vi "Plot Multi-XY_modded.vi"(0 "picture":picture, 1 "desired font(Application)":T6(ring)=enum."Application Font", 3 "[user-specified font]":T7, 5 "data":cluster{"data":cluster{"x":dbl, "y":dbl}[]}[](array[cluster]) {"data"."y" format="%0.2f"; "data"."x" format="%0.2f"}, 7 "dimensions (w,h)":cluster{"width":i16, "height":i16}, 9 "line style":T1={"Width"=1, "Style"=enum."Solid"}, 11 "top left point(0, 0)":cluster{"x":i16, "y":i16}, 12 "cartesian axis attributes":T8={"x minimum"=0.0, "x maximum"=0.0, "x log?"=FALSE, "x precision"=1, "x format"=enum."Decimal", "y minimum"=0.0, "y maximum"=0.0, "y log?"=FALSE, "y precision"=1, "y format"=enum."Decimal"} {"x minimum" format="%0.2f"; "x maximum" format="%0.2f"; "y minimum" format="%0.2f"; "y maximum" format="%0.2f"}, 13 "cartesian grid cosmetics":T3={"line color"=39168, "text color"=65280, "tick length(3)"=3, "crossing axes"=FALSE, "visible grid?"=TRUE}, 14 "XY plot cosmetics":T5(array[cluster])=[{"plot color"=16776960, "XY plot type"=enum."sized scatter plot", "baseline"=0.0}, {"plot color"=65280, "XY plot type"=enum."connected points", "baseline"=0.0}, {"plot color"=65535, "XY plot type"=enum."connected points", "baseline"=0.0}] {"baseline" format="%0.2f"}, 15 "[sized scatter plot cosmetics]":T2(array[cluster])=[{"min size"=1, "max size"=5, "maps to max size"=5, "color array"=[16776960, 65280, 16711680, 255]}]) -> (4 "new picture":picture)   [LabVIEW 2018]
doc: "Takes a picture and an array of plots and appends a picture of an XY graph of the data with the plots overlaid on the same graph."
uses:
  <vilib>/picture/cartesn2.llb/XY Plot Type.ctl
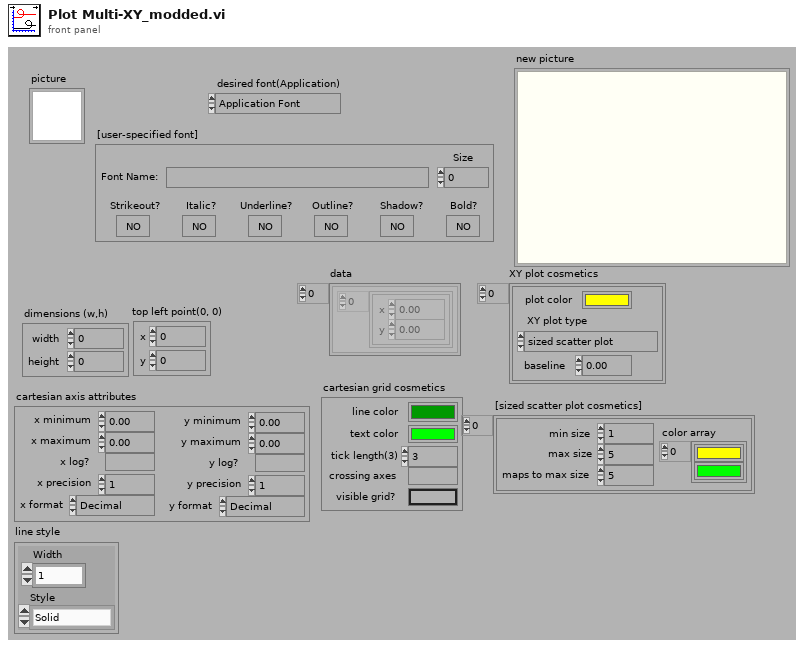
[diagram p1: front panel]
types:
  T1 = cluster{"Width":u16, "Style":enum32{"Solid", "Dash", "Dot", "DashDot", "DashDotDot"}}
  T2 = cluster{"min size":i16, "max size":i16, "maps to max size":i16, "color array":u32[]}[]
  T3 = cluster{"line color":u32, "text color":u32, "tick length(3)":i16, "crossing axes":bool, "visible grid?":bool}
  T4 = typedef "XY Plot Type.ctl" = enum16{"points", "squares", "circles", "connected points", "connected squares", "connected circles", "comb plot", "sized scatter plot", "sized-colored scatter plot", "min-max lines"}
  T5 = cluster{"plot color":u32, "XY plot type":T4, "baseline":dbl}[]
  T6 = enum16{"User-specified Font", "Application Font", "System Font", "Dialog Font"}
  T7 = cluster{"Font Name:":string, "Size":i16, "Strikeout?":bool, "Italic?":bool, "Underline?":bool, "Outline?":bool, "Shadow?":bool, "Bold?":bool}
  T8 = cluster{"x minimum":dbl, "x maximum":dbl, "x log?":bool, "x precision":u8, "x format":enum8{"Decimal", "Scientific", "Engineering", "Binary", "Octal", "Hex", "Timestamp"}, "y minimum":dbl, "y maximum":dbl, "y log?":bool, "y precision":u8, "y format":enum8{"Decimal", "Scientific", "Engineering", "Binary", "Octal", "Hex", "Timestamp"}}
  T9 = cluster{"left":i16, "top":i16, "right":i16, "bottom":i16}
  T10 = cluster{"plot color":u32, "XY plot type":T4, "baseline":dbl}
  T11 = cluster{"min size":i16, "max size":i16, "maps to max size":i16, "color array":u32[]}
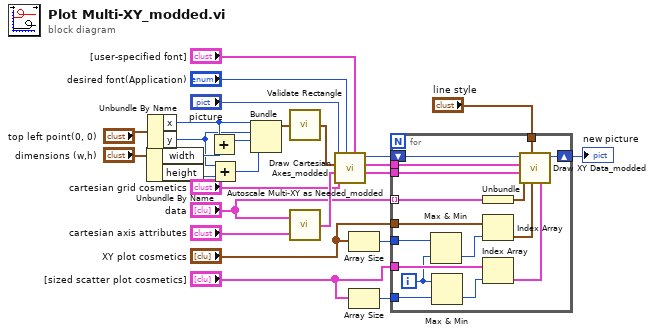
[diagram p0: block diagram]
diagram:
  n1 = Unbundle By Name("dimensions (w,h)") -> ("width"=w10:i16, "height"=w9:i16)
  n2 = Unbundle By Name("top left point(0, 0)") -> ("x"=w8:i16, "y"=w7:i16)
  n3 = Add(x=w8, y=w10) -> (x+y=w6:i16)
  n4 = Add(x=w7, y=w9) -> (x+y=w5:i16)
  n5 = Bundle("x"=w8, "y"=w7, w6, w5) -> (w2:cluster{"x":i16, "y":i16, i16, i16})  [unwired: 1 in]
  n6 = call <vilib>:"Validate Rectangle.vi"("rect"=w2) -> ("valid rect"=w18:T9)
  n7 = call "Autoscale Multi-XY as Needed_modded.vi"("axis attributes"="cartesian axis attributes", "multi-xy data"="data") -> ("axis attributes"=w26:T8)
  n8 = call "Draw Cartesian Axes_modded.vi"("[user-specified font]"="[user-specified font]", "desired font(Application)"="desired font(Application)", "grid cosmetics"="cartesian grid cosmetics", "axis attributes"=w26, "bounding rect"=w18, "picture"="picture") -> ("y scale factors"=w19:cluster{"a":dbl, "b":dbl, "log?":bool}, "x scale factors"=w20:cluster{"a":dbl, "b":dbl, "log?":bool}, "new picture"=w23:picture)  [unwired: 3 in]
  n9 = Array Size(array="XY plot cosmetics") -> (size(s)=w11:i32)
  n10 = Array Size(array="[sized scatter plot cosmetics]") -> (size(s)=w13:i32)
  n11 = for {
    shift-right: [w39] -> w22
    shift-left: w23 -> [w40]
    tunnel: w19 -> [w42]
    tunnel: w20 -> [w41]
    tunnel: "XY plot cosmetics" -> [w38]
    tunnel: "data" -> [w37] mode=indexing
    tunnel: "[sized scatter plot cosmetics]" -> [w34]
    tunnel: w13 -> [w32]
    tunnel: w11 -> [w29]
    tunnel: "line style" -> [w27]
    i -> [w28]
    n12 = Max & Min(x=w29, y=w28) -> (min(x,y)=w30:i32)  [unwired: 1 out]
    n13 = Max & Min(x=w28, y=w32) -> (min(x,y)=w31:i32)  [unwired: 1 out]
    n14 = Unbundle(w37) -> ("data"=w36:cluster{"x":dbl, "y":dbl}[])
    n15 = Index Array(array=w38, index=w30) -> (element=w35:T10)
    n16 = Index Array(array=w34, index=w31) -> (element=w33:T11)
    n17 = call "Draw XY Data_modded.vi"("[sized scatter plot cosmetics]"=w33, "xy cosmetics"=w35, "pen"=w27, "xy data"=w36, "y scale factors"=w42, "x scale factors"=w41, "picture"=w40) -> ("new picture"=w39:picture)  [unwired: 4 in]
  }
  "new picture" <- w22
